vi "imp_test_v9_1.vi"() -> ()   [LabVIEW 2014]
uses:
  <vilib>/LabVIEW Targets/FPGA/cRIO/shared/nicrio_ModuleControls/nicrio_cRIO-9237_DataRatesRing.ctl
  <vilib>/LabVIEW Targets/FPGA/cRIO/shared/nicrio_ModuleControls/nicrio_cRIO-9237_ExcitationVoltageRing.ctl
  <vilib>/rvi/FXPMathLib/FxpSinAndCos/subVIs/nifxpmath_SinAndCos_SimConfig.ctl
  <vilib>/rvi/Emulation/niFpgaGetClockAttributes.vi
  <vilib>/rvi/Emulation/niFpgaSctlEmulationGetInTimedLoop.vi
  <vilib>/rvi/Emulation/niFpgaEmulationReportErrorSimple.vi
  <vilib>/rvi/Emulation/niFpgaProcessEmulError.vi
  <vilib>/rvi/interface/RandomDataEmulation/nirviRandomDataMultiElementFPGAFIFO.vi
  <instcachedir>/0/nirviRandomDataMultiElementFPGAFIFO_AD0CFC12EF974623A9C2E4184BC062B2.lvgen/nirviRandomDataMultiElementFPGAFIFO_AD0CFC12EF974623A9C2E4184BC062B2_025.vi
  <vilib>/rvi/interface/RandomDataEmulation/niFpgaRandomDataHandleErrors.vi
  <vilib>/rvi/Emulation/niFpgaCriticalErrorInLSC.vi
  <vilib>/rvi/FXPMathLib/FxpSinAndCos/simVIs/DllFxpSinAndCosTemp_sub.vi
  <vilib>/rvi/eio/common/nirviEmuTemplateMethod_errors.vi
  <vilib>/rvi/eio/common/nirviEmuTemplatePropertySet_errors.vi
  <vilib>/rvi/DataTransferAndStorage/Container/XNode/niFpgaContainer.xnode
  <vilib>/rvi/interface/RandomDataEmulation/nirviRandomDataFpgaMultiElementTemplate.vi
  <vilib>/rvi/FXPMathLib/FxpMul/XNode/nifxpmath_Multiplier.xnode
  <vilib>/rvi/FXPMathLib/FxpSinAndCos/XNode/nifxpmath_SinAndCos.xnode
  <vilib>/eio/EIONode/EIONode.xnode
  <vilib>/rvi/Analysis/measure/butterworth/XNode/niFpgaButterworthFilter.xnode
  <vilib>/rvi/FXPMathLib/FxpSub/XNode/nifxpmath_Sub.xnode
  <vilib>/rvi/FXPMathLib/FxpAdd/XNode/nifxpmath_Add.xnode
  <vilib>/eio/EIOPropertyNode/EIOPropertyNode.xnode
  <vilib>/rvi/eio/common/nirviEmuTemplatePropertyGet_errors.vi
  <vilib>/rvi/eio/common/nirviEmuTemplatePropertyGet_noerrors.vi
  <vilib>/rvi/eio/common/nirviEmuTemplatePropertySet_noerrors.vi
  <vilib>/rvi/FXPMathLib/sim/FxpSim.dll
panel:
  in  "Set 6":bool
  in  "Set 5":bool
  in  "Set 4":bool
  in  "Set 3":bool
  in  "Set 2":bool
  in  "Set 1":bool
  out "Dy1_d (T)":fxp<+/-,56,14>
  out "omega_y1 (T)":fxp<+/-,36,13>
  out "Dp1_d (T)":fxp<+/-,36,13>
  out "omega_p1 (T)":fxp<+/-,36,13>
  out "Dy2_d (T)":fxp<+/-,36,13>
  out "Dp2_d (T)":fxp<+/-,36,13>
  out "omega_y2 (T)":fxp<+/-,36,13>
  out "omega_p2 (T)":fxp<+/-,36,13>
  out "mt_omega_y2":u32
  out "mt_omega_p2":u32
  out "rad_y2":fxp<+/-,33,20>
  out "D_y2":fxp<+/-,32,7>
  out "rad_y1":fxp<+/-,33,20>
  out "D_y1":fxp<+/-,32,7>
  out "Encoder Position_y1":i32
  out "Encoder Position_y2":i32
  out "Encoder Position_p2":i32
  out "D_p2":fxp<+/-,32,7>
  out "rad_p2":fxp<+/-,33,20>
  out "D_p1":fxp<+/-,32,7>
  out "rad_p1":fxp<+/-,33,20>
  out "Encoder Position_p1":i32
  in  "Mag. factor_y":fxp<+/-,20,3>
  in  "Mag. encoder_y":bool
  out "omega_y (rad/s)":fxp<+/-,36,13>
  out "Dy_d (mm/s)":fxp<+/-,36,13>
  in  "Vy. Est.":i16(ring) items=["T", "Mavg"]
  out "omega_y (Mavg)":fxp<+/-,36,14>
  out "Dy_d (Mavg)":fxp<+/-,36,14>
  in  "Dy_d_M_avg_Tc (uSec)":i32
  out "Dp_d (Mavg)":fxp<+/-,36,14>
  out "omega_p (Mavg)":fxp<+/-,36,14>
  in  "Dp_d_M_avg_Tc (uSec)":i32
  out "Dp_d (T)":fxp<+/-,36,13>
  out "omega_p (T)":fxp<+/-,36,13>
  in  "Vp. Est.":i16(ring) items=["T", "Mavg"]
  in  "Mag. factor_p":fxp<+/-,20,3>
  in  "Mag. encoder_p":bool
  in  "Belt_out_p":fxp<+/-,7,7>
  in  "Belt_in_p":fxp<+/-,6,6>
  in  "Belt_out_y":fxp<+/-,7,7>
  in  "Belt_in_y":fxp<+/-,6,6>
  out "Fp_dc":fxp<+/-,32,10>
  out "Fy_dc":fxp<+/-,32,10>
  in  "Zero_y":bool
  in  "Zero_p":bool
  in  "mt0_omega_p":u32
  in  "Encoder reset":bool
  out "fpt_d":fxp<+/-,36,18>
  out "Dp_error_dd":fxp<+/-,36,16>
  out "Dp_error_d":fxp<+/-,33,8>
  in  "Dp_dd coeff.":i32[](array[numeric])=[946630756, 63555534]
  out "Dp_dd":fxp<+/-,36,25>
  out "dFp_PID":fxp<+/-,36,18>
  in  "dFp_PID coeff.":i32[](array[numeric])=[946630756, 63555534]
  out "fpt_i":fxp<+/-,34,18>
  in  "Bv_p":fxp<+/-,22,8>
  in  "Kv_p":fxp<+/-,22,8>
  out "Dp_error":fxp<+/-,22,7>
  out "Dpr_sin":fxp<+/-,22,7>
  in  "Sin offset_p":fxp<+/-,22,7>
  in  "Sin magnitude_p":fxp<+/-,21,6>
  out "Dpr_sin_dd":fxp<+/-,35,20>
  out "Dpr_sin_d":fxp<+/-,33,15>
  out "Sin omega_p":fxp<+/-,34,9>
  in  "Sin wave freq._p (Hz)":fxp<+/-,32,6>
  in  "Dpr_step":fxp<+/-,22,7>
  out "Dpr_for":fxp<+/-,22,7>
  in  "Command_p":i16(ring) items=["Step", "Sine"]
  in  "Ki_p":fxp<+/-,36,9>
  out "Fp_PID":fxp<+/-,36,16>
  in  "fp_tolorance":fxp<+,22,6>
  out "fp_tilde":fxp<+/-,33,10>
  in  "Kd_p":fxp<+/-,36,9>
  in  "Kp_p":fxp<+/-,36,9>
  out "Fr_p":fxp<+/-,32,10>
  in  "S/F coeff_p":fxp<+/-,25,-10>
  in  "S/F coeff_y":fxp<+/-,25,-10>
  out "va_p":fxp<+/-,36,7>
  out "vb_p":fxp<+/-,37,8>
  out "vq_p_F":fxp<+/-,20,5> format="%.57g"
  out "vd_p_F":fxp<+/-,20,5>
  in  "dFp_add":bool
  in  "Stop motor_p":bool
  out "Force_p":fxp<+/-,32,10>
  in  "Strain selection_p":i16(ring) items=["Raw", "Avg.8", "Avg.8 w. filter"]
  out "Strain_p (Avg8 w. f)":fxp<+/-,36,8>
  in  "Strain_p Avg.8 coeff.":i32[](array[numeric])=[946630756, 63555534]
  out "Strain_p (Avg8)":fxp<+/-,36,4>
  out "Raw Strain_p":fxp<+/-,36,4>
  out "Mod6/AI3":fxp<+/-,36,4>
  in  "Strain gage reset_p":bool
  out "Dp_d (mm/s)":fxp<+/-,36,13>
  out "omega_p (rad/s)":fxp<+/-,36,13>
  out "mt_omega_p1":u32
  out "rad_p(NrTheta)":fxp<+/-,33,20>
  out "D_p(mm)":fxp<+/-,32,7>
  out "Encoder Position_p":i32
  in  "Encoder reset_p":bool
  out "Strain_y (Avg8 w. f)":fxp<+/-,36,8>
  in  "Strain_y Avg8 coeff.":i32[](array[numeric])=[-898916953, 1957103773, 3888751]
  out "Dyr_for":fxp<+/-,22,7>
  in  "Command_y":i16(ring) items=["Step", "Sine"]
  out "Strain_y (Avg8)":fxp<+/-,36,4>
  in  "Strain selection_y":i16(ring) items=["Raw", "Avg.8", "Avg.8 w. filter"]
  out "vb_y":fxp<+/-,38,8>
  out "va_y":fxp<+/-,38,8>
  out "fyt_d":fxp<+/-,36,18>
  out "Fr_y":fxp<+/-,32,10>
  in  "Bv_y":fxp<+/-,22,8>
  out "Dy_error_dd":fxp<+/-,36,16>
  out "Dy_error_d":fxp<+/-,33,8>
  in  "Kv_y":fxp<+/-,22,8>
  out "Dy_error":fxp<+/-,22,7>
  out "Dyr_sin_dd":fxp<+/-,35,20>
  out "Dyr_sin_d":fxp<+/-,33,15>
  out "Sin omega_y":fxp<+/-,34,9>
  out "Dyr_sin":fxp<+/-,22,7>
  in  "Sin offset_y":fxp<+/-,22,7>
  in  "Sin magnitude_y":fxp<+/-,21,6>
  out "Time now(s)":fxp<+,52,14>
  in  "Sin wave freq._y (Hz)":fxp<+/-,32,6>
  in  "Dyr_step":fxp<+/-,22,7>
  in  "Drive mode":i16(ring) items=["Backward", "Forward"]
  out "Dy_dd":fxp<+/-,36,25>
  in  "Dy_dd coeff.":i32[](array[numeric])=[946630756, 63555534]
  out "dFy_PID":fxp<+/-,36,18>
  in  "dFy_PID coeff.":i32[](array[numeric])=[946630756, 63555534]
  out "fyt_i":fxp<+/-,36,16>
  out "Fy_PID":fxp<+/-,36,16>
  in  "fy_tolorance":fxp<+,22,6>
  in  "Ki_y":fxp<+/-,36,9>
  in  "Kd_y":fxp<+/-,36,9>
  out "fy_tilde":fxp<+/-,32,10>
  in  "Kp_y":fxp<+/-,36,9>
  out "vq_y_F":fxp<+/-,20,5> format="%.57g"
  out "vd_y_F":fxp<+/-,20,5>
  in  "dFy_add":bool
  in  "Stop motor_y":bool
  out "Dy_d (T)":fxp<+/-,36,13>
  out "omega_y (T)":fxp<+/-,36,13>
  in  "mt0_omega_y":u32
  out "mt_omega_y1":u32
  out "rad_y(NrTheta)":fxp<+/-,33,20>
  out "D_y(mm)":fxp<+/-,32,7>
  out "Encoder Position_y":i32
  in  "Encoder reset_y":bool
  in  "Ini coe.":bool
  out "Loop rate (kHz)":fxp<+/-,36,7>
  out "Force_y":fxp<+/-,32,10>
  out "Raw Strain_y":fxp<+/-,36,4>
  in  "Strain gage reset_y":bool
  in  "Stop (Strain)":bool
  out "Mod6/AI2":fxp<+/-,36,4>
  in  "Excitation Voltage":T1 items=["2.5 Volts", "3.3 Volts", "5.0 Volts", "10.0 Volts", "External Excitation"]
  in  "Data Rate":T2=1 items=["50.000 kS/s (NI 9237)"=1, "25.000 kS/s (NI 9237)"=2, "16.667 kS/s (NI 9237)"=3, "12.500 kS/s (NI 9237)"=4, "10.000 kS/s (NI 9237)"=5, "8.333 kS/s (NI 9237)"=6, "7.143 kS/s (NI 9237)"=7, "6.250 kS/s (NI 9237)"=8, "5.556 kS/s (NI 9237)"=9, "5.000 kS/s (NI 9237)"=10, "4.545 kS/s (NI 9237)"=11, "4.167 kS/s (NI 9237)"=12, "3.846 kS/s (NI 9237)"=13, "3.571 kS/s (NI 9237)"=14, "3.333 kS/s (NI 9237)"=15, "3.125 kS/s (NI 9237)"=16, "2.941 kS/s (NI 9237)"=17, "2.778 kS/s (NI 9237)"=18, "2.632 kS/s (NI 9237)"=19, "2.500 kS/s (NI 9237)"=20, "2.381 kS/s (NI 9237)"=21, "2.273 kS/s (NI 9237)"=22, "2.174 kS/s (NI 9237)"=23, "2.083 kS/s (NI 9237)"=24, "2.000 kS/s (NI 9237)"=25, "1.923 kS/s (NI 9237)"=26, "1.852 kS/s (NI 9237)"=27, "1.786 kS/s (NI 9237)"=28, "1.724 kS/s (NI 9237)"=29, "1.667 kS/s (NI 9237)"=30, "1.613 kS/s (NI 9237)"=31]
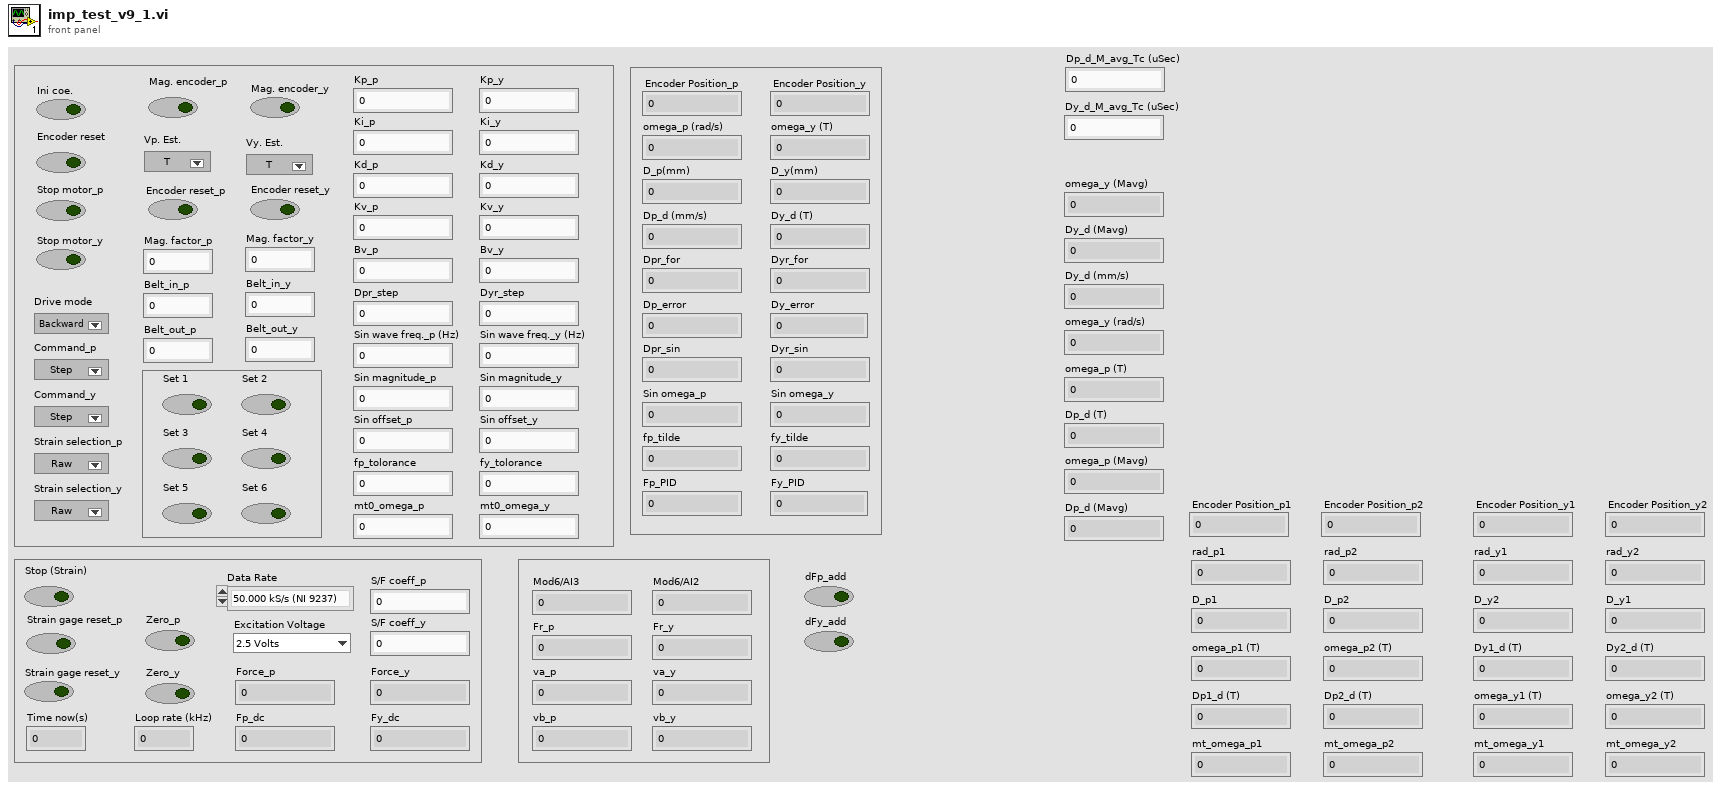
[diagram p1: front panel]
types:
  T1 = typedef "nicrio_cRIO-9237_ExcitationVoltageRing.ctl" = u8
  T2 = typedef "nicrio_cRIO-9237_DataRatesRing.ctl" = u8
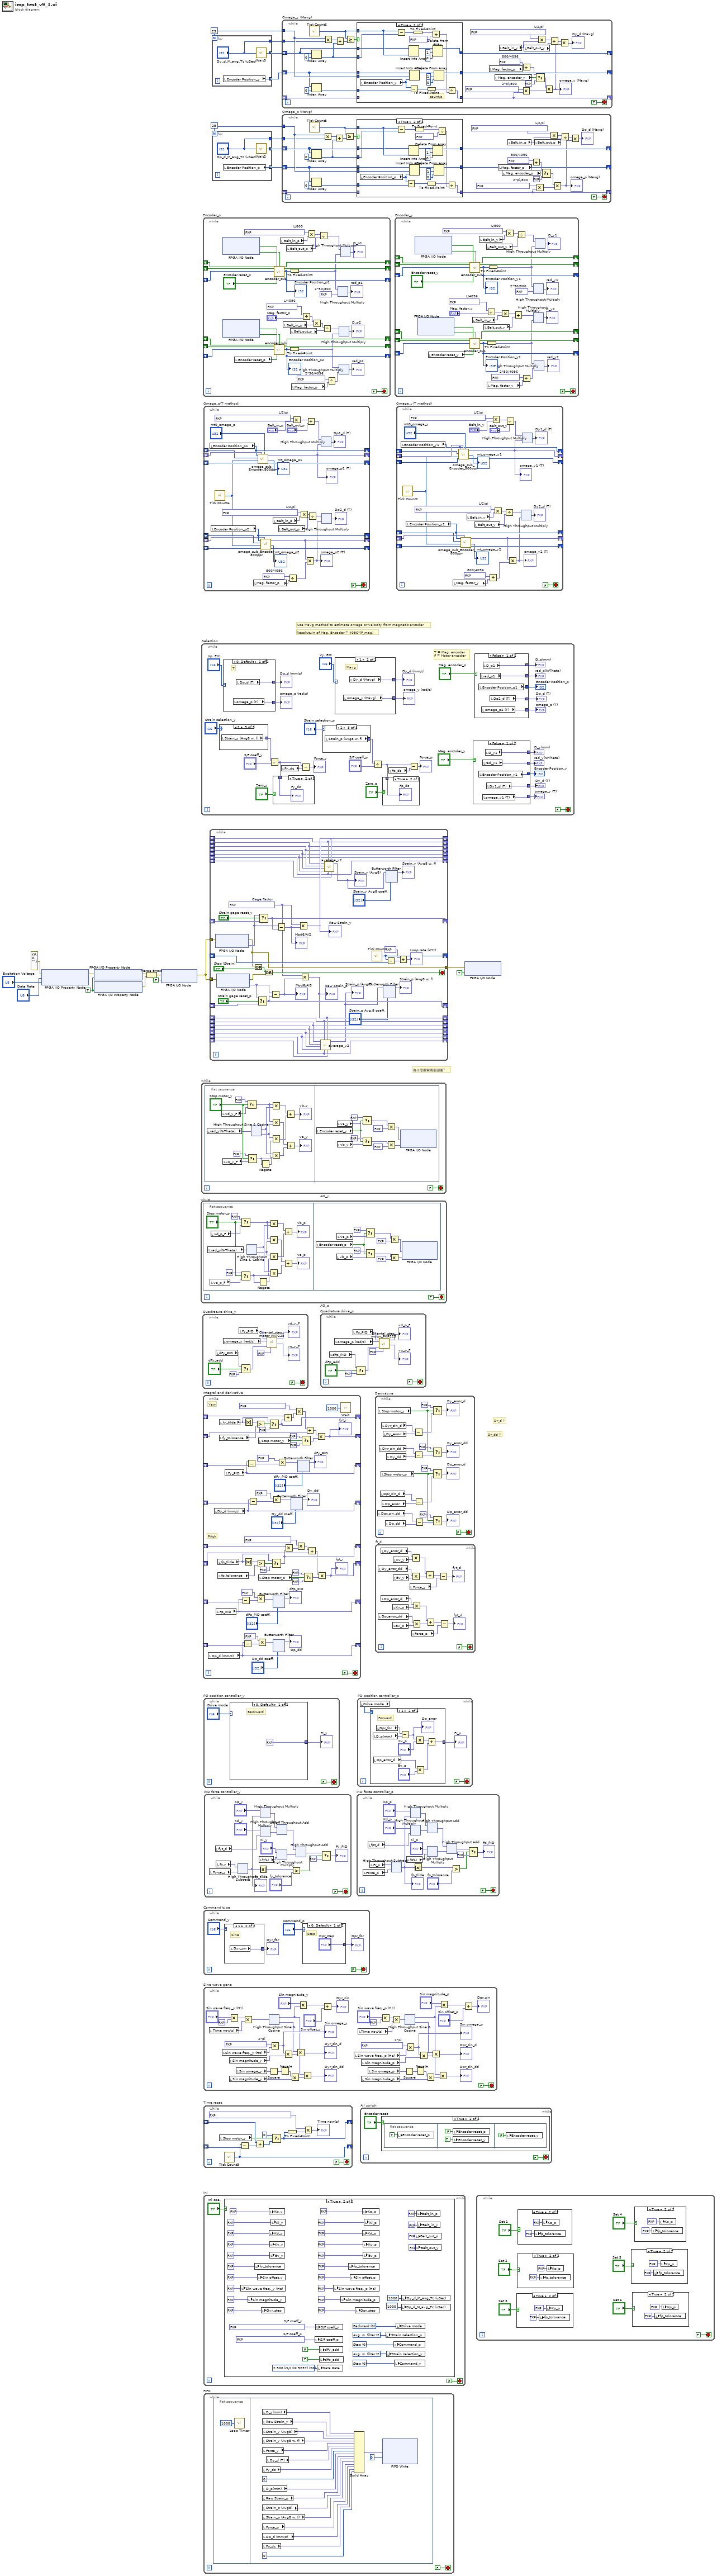
[diagram p0: block diagram]
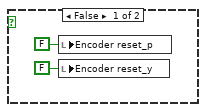
[diagram p10: hidden frame]
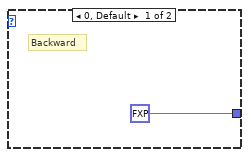
[diagram p11: hidden frame]
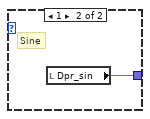
[diagram p12: hidden frame]
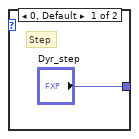
[diagram p13: hidden frame]
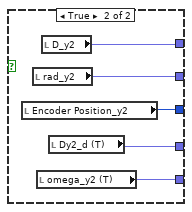
[diagram p14: hidden frame]
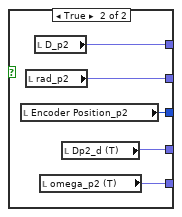
[diagram p15: hidden frame]
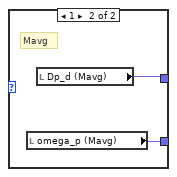
[diagram p16: hidden frame]
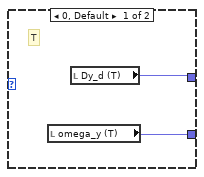
[diagram p17: hidden frame]
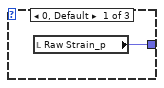
[diagram p20: hidden frame]
diagram:
  w5 = 25
  w8 = 25
  w13 = TRUE ("Half-Bridge Enable")
  # "Resolutuin of Mag. Encoder = 4096*(F_mag)"
  # "use Mavg method to estimate omega or velocity from magnetic encoder"
  # "為什麼要寫兩個迴圈?"
  # "Dr_dd ?"
  # "Dr_d ?"
  n1 = xnode "FPGA I/O Property Node"("error in"=errorcluster {"status"=FALSE, "code"=0, "source"=""}, "Data Rate"="Data Rate", "Excitation Voltage"="Excitation Voltage") -> ("error out"=w18:errorcluster)  [unwired: 1 in, 1 out]
  n2 = xnode "FPGA I/O Property Node"("error in"=w18, "Half-Bridge Enable"=w13) -> ("error out"=w11:errorcluster)  [unwired: 1 in, 1 out]
  n3 = xnode "FPGA I/O Property Node"("Half-Bridge Enable"=w13) -> ("error out"=w10:errorcluster)  [unwired: 2 in, 1 out]
  n4 = Merge Errors(w11, w10) -> (w12:errorcluster)
  n5 = xnode "FPGA I/O Node"("error in"=w12, "Mod6/Start"=TRUE) -> ("error out"=w16:errorcluster)  [unwired: 1 in, 1 out]
  n6 = while "AO_p" {
    stop <- FALSE stop-if-true
    n7 = flat-sequence {
      frame #0 {
        n8 = local read "rad_p(NrTheta)"() -> (w33:fxp<+/-,33,20>)
        n9 = local read "vq_p_F"() -> (w34:fxp<+/-,20,5>)
        n10 = local read "vd_p_F"() -> (w36:fxp<+/-,20,5>)
        n11 = Select(t=fxp<+/-,20,5> 0.0, s="Stop motor_p", f=w36) -> (s? t:f=w25:fxp<+/-,20,5>)
        n12 = Select(t=fxp<+,1,1> 0.0, s="Stop motor_p", f=w34) -> (s? t:f=w24:fxp<+/-,20,5>)
        n13 = xnode "High Throughput Sine & Cosine"("x (pi)"=w33) -> ("sin(x)"=w27:fxp<+/-,16,2>, "cos(x)"=w26:fxp<+/-,16,2>)
        n14 = Negate(x=w24) -> (-x=w32:fxp<+/-,21,6>)
        n15 = Multiply(x=w25, y=w27) -> (x*y=w31:fxp<+/-,36,7>)
        n16 = Multiply(x=w25, y=w26) -> (x*y=w29:fxp<+/-,36,7>)
        n17 = Multiply(x=w26, y=w24) -> (x*y=w30:fxp<+/-,36,7>)
        n18 = Multiply(x=w27, y=w32) -> (x*y=w28:fxp<+/-,35,6>)
        n19 = Add(x=w31, y=w30) -> (x+y=→"vb_p":fxp<+/-,37,8>)
        n20 = Add(x=w29, y=w28) -> (x+y=→"va_p":fxp<+/-,36,7>)
      }
      frame #1 {
        n21 = local read "Encoder reset_p"() -> (w69:bool)
        n22 = local read "vb_p"() -> (w70:fxp<+/-,37,8>)
        n23 = local read "va_p"() -> (w71:fxp<+/-,36,7>)
        n24 = Select(t=fxp<+,2,2> 3.0, s=w69, f=w71) -> (s? t:f=w77:fxp<+/-,36,7>)
        n25 = Select(t=fxp<+,1,1> 0.0, s=w69, f=w70) -> (s? t:f=w76:fxp<+/-,37,8>)
        n26 = Multiply(x=w77, y=fxp<+/-,1,0> -0.5) -> (x*y=w72:fxp<+/-,36,6>)
        n27 = Multiply(x=w76, y=fxp<+/-,1,0> -0.5) -> (x*y=w73:fxp<+/-,36,6>)
        n28 = xnode "FPGA I/O Node"("Mod8/AO0"=w72, "Mod8/AO1"=w73) -> ()  [unwired: 2 in, 2 out]
      }
    }
  }
  n29 = while "AO_y" {
    stop <- FALSE stop-if-true
    n30 = flat-sequence {
      frame #0 {
        n31 = local read "rad_y(NrTheta)"() -> (w97:fxp<+/-,33,20>)
        n32 = local read "vd_y_F"() -> (w95:fxp<+/-,20,5>)
        n33 = local read "vq_y_F"() -> (w94:fxp<+/-,20,5>)
        n34 = Select(t=fxp<+/-,20,5> 0.0, s="Stop motor_y", f=w95) -> (s? t:f=w89:fxp<+/-,20,5>)
        n35 = Select(t=fxp<+/-,20,5> 0.0, s="Stop motor_y", f=w94) -> (s? t:f=w88:fxp<+/-,20,5>)
        n36 = xnode "High Throughput Sine & Cosine"("x (pi)"=w97) -> ("sin(x)"=w91:fxp<+/-,17,2>, "cos(x)"=w90:fxp<+/-,17,2>)
        n37 = Negate(x=w88) -> (-x=w87:fxp<+/-,21,6>)
        n38 = Multiply(x=w89, y=w91) -> (x*y=w86:fxp<+/-,37,7>)
        n39 = Multiply(x=w89, y=w90) -> (x*y=w84:fxp<+/-,37,7>)
        n40 = Multiply(x=w90, y=w88) -> (x*y=w85:fxp<+/-,37,7>)
        n41 = Multiply(x=w91, y=w87) -> (x*y=w83:fxp<+/-,36,6>)
        n42 = Add(x=w86, y=w85) -> (x+y=→"vb_y":fxp<+/-,38,8>)
        n43 = Add(x=w84, y=w83) -> (x+y=→"va_y":fxp<+/-,37,7>)
      }
      frame #1 {
        n44 = local read "Encoder reset_y"() -> (w130:bool)
        n45 = local read "va_y"() -> (w129:fxp<+/-,38,8>)
        n46 = local read "vb_y"() -> (w128:fxp<+/-,38,8>)
        n47 = Select(t=fxp<+,2,2> 3.0, s=w130, f=w129) -> (s? t:f=w134:fxp<+/-,38,8>)
        n48 = Select(t=fxp<+,1,1> 0.0, s=w130, f=w128) -> (s? t:f=w133:fxp<+/-,38,8>)
        n49 = Multiply(x=w134, y=fxp<+/-,1,0> -0.5) -> (x*y=w137:fxp<+/-,39,8>)
        n50 = Multiply(x=w133, y=fxp<+/-,1,0> -0.5) -> (x*y=w138:fxp<+/-,37,6>)
        n51 = xnode "FPGA I/O Node"("Mod8/AO2"=w137, "Mod8/AO3"=w138) -> ()  [unwired: 2 in, 2 out]
      }
    }
  }
  n52 = while "Selection" {
    stop <- FALSE stop-if-true
    # "T = Mag. encoder\nF = Motor encoder"
    n53 = case shown="2" "Strain selection_y" {
      tunnel: [w205 w206 w207] -> w170
      frame 0, Default {
        n54 = local read "Raw Strain_y"() -> (w205:fxp<+/-,36,4>)
      }
      frame 1 {
        n55 = local read "Strain_y (Avg8)"() -> (w206:fxp<+/-,36,4>)
      }
      frame 2 {
        n56 = local read "Strain_y (Avg8 w. f)"() -> (w207:fxp<+/-,36,8>)
      }
    }
    n57 = case shown="0, Default" "Vp. Est." {
      tunnel: [w193 w194] -> w153
      tunnel: [w192 w195] -> w154
      frame 0, Default {
        # "T"
        n58 = local read "omega_p (T)"() -> (w193:fxp<+/-,36,13>)
        n59 = local read "Dp_d (T)"() -> (w192:fxp<+/-,36,13>)
      }
      frame 1 {
        # "Mavg"
        n60 = local read "omega_p (Mavg)"() -> (w194:fxp<+/-,36,14>)
        n61 = local read "Dp_d (Mavg)"() -> (w195:fxp<+/-,36,14>)
      }
    }
    "Dp_d (mm/s)" <- w154
    "omega_p (rad/s)" <- w153
    n62 = Divide(x=w170, y="S/F coeff_y") -> (x/y=w163:fxp<+/-,32,10>)
    n63 = case shown="True" "Zero_y" {
      tunnel: w163 -> [_ w201]
      frame False {
      }
      frame True {
        "Fy_dc" <- w201
      }
    }
    n64 = local read "Fy_dc"() -> (w164:fxp<+/-,32,10>)
    n65 = Subtract(x=w163, y=w164) -> (x-y=→"Force_y":fxp<+/-,33,11>)
    n66 = case shown="2" "Strain selection_p" {
      tunnel: [w202 w203 w204] -> w168
      frame 0, Default {
        n67 = local read "Raw Strain_p"() -> (w202:fxp<+/-,36,4>)
      }
      frame 1 {
        n68 = local read "Strain_p (Avg8)"() -> (w203:fxp<+/-,36,4>)
      }
      frame 2 {
        n69 = local read "Strain_p (Avg8 w. f)"() -> (w204:fxp<+/-,36,8>)
      }
    }
    n70 = case shown="1" "Vy. Est." {
      tunnel: [w197 w199] -> w156
      tunnel: [w196 w198] -> w157
      frame 0, Default {
        # "T"
        n71 = local read "omega_y (T)"() -> (w196:fxp<+/-,36,13>)
        n72 = local read "Dy_d (T)"() -> (w197:fxp<+/-,36,13>)
      }
      frame 1 {
        # "Mavg"
        n73 = local read "omega_y (Mavg)"() -> (w198:fxp<+/-,36,14>)
        n74 = local read "Dy_d (Mavg)"() -> (w199:fxp<+/-,36,14>)
      }
    }
    "Dy_d (mm/s)" <- w156
    "omega_y (rad/s)" <- w157
    n75 = Divide(x=w168, y="S/F coeff_p") -> (x/y=w160:fxp<+/-,32,10>)
    n76 = case shown="True" "Zero_p" {
      tunnel: w160 -> [_ w200]
      frame False {
      }
      frame True {
        "Fp_dc" <- w200
      }
    }
    n77 = local read "Fp_dc"() -> (w158:fxp<+/-,32,10>)
    n78 = Subtract(x=w160, y=w158) -> (x-y=→"Force_p":fxp<+/-,33,11>)
    n79 = case shown="False" "Mag. encoder_y" {
      tunnel: [w176 w180] -> w144
      tunnel: [w175 w181] -> w145
      tunnel: [w174 w179] -> w147
      tunnel: [w172 w178] -> w141
      tunnel: [w173 w177] -> w140
      frame False {
        n80 = local read "Encoder Position_y1"() -> (w174:i32)
        n81 = local read "rad_y1"() -> (w176:fxp<+/-,33,20>)
        n82 = local read "omega_y1 (T)"() -> (w172:fxp<+/-,36,13>)
        n83 = local read "D_y1"() -> (w175:fxp<+/-,32,7>)
        n84 = local read "Dy1_d (T)"() -> (w173:fxp<+/-,56,14>)
      }
      frame True {
        n85 = local read "Encoder Position_y2"() -> (w179:i32)
        n86 = local read "rad_y2"() -> (w180:fxp<+/-,33,20>)
        n87 = local read "omega_y2 (T)"() -> (w178:fxp<+/-,36,13>)
        n88 = local read "D_y2"() -> (w181:fxp<+/-,32,7>)
        n89 = local read "Dy2_d (T)"() -> (w177:fxp<+/-,36,13>)
      }
    }
    "D_y(mm)" <- w145
    "rad_y(NrTheta)" <- w144
    "Encoder Position_y" <- w147
    "Dy_d (T)" <- w140
    "omega_y (T)" <- w141
    n90 = case shown="False" "Mag. encoder_p" {
      tunnel: [w186 w191] -> w149
      tunnel: [w185 w190] -> w150
      tunnel: [w184 w189] -> w151
      tunnel: [w182 w188] -> w143
      tunnel: [w183 w187] -> w142
      frame False {
        n91 = local read "Encoder Position_p1"() -> (w184:i32)
        n92 = local read "rad_p1"() -> (w185:fxp<+/-,33,20>)
        n93 = local read "omega_p2 (T)"() -> (w182:fxp<+/-,36,13>)
        n94 = local read "D_p1"() -> (w186:fxp<+/-,32,7>)
        n95 = local read "Dp2_d (T)"() -> (w183:fxp<+/-,36,13>)
      }
      frame True {
        n96 = local read "Encoder Position_p2"() -> (w189:i32)
        n97 = local read "rad_p2"() -> (w190:fxp<+/-,33,20>)
        n98 = local read "D_p2"() -> (w191:fxp<+/-,32,7>)
        n99 = local read "omega_p2 (T)"() -> (w188:fxp<+/-,36,13>)
        n100 = local read "Dp2_d (T)"() -> (w187:fxp<+/-,36,13>)
      }
    }
    "D_p(mm)" <- w149
    "rad_p(NrTheta)" <- w150
    "Encoder Position_p" <- w151
    "Dp_d (T)" <- w142
    "omega_p (T)" <- w143
  }
  n101 = while "Quadrature drive_y" {
    stop <- FALSE stop-if-true
    n102 = local read "dFy_PID"() -> (w209:fxp<+/-,36,18>)
    n103 = local read "omega_y (rad/s)"() -> (w217:fxp<+/-,36,13>)
    n104 = local read "Fy_PID"() -> (w210:fxp<+/-,36,16>)
    n105 = Select(t=w209, s="dFy_add", f=fxp<+,1,1> 0.0) -> (s? t:f=w213:fxp<+/-,36,18>)
    n106 = call "Oriental_step_motor_PKP225.vi"("F_Threshold"=fxp<+,12,12> 10.0, "dFmr"=w213, "omega"=w217, "Fmr"=w210) -> ("vq_F"=→"vq_y_F":fxp<+/-,20,5>, "vd_F"=→"vd_y_F":fxp<+/-,20,5>)  [unwired: 6 in]
  }
  n107 = while "Encoder_p" {
    shift-right: [w255] -> _
    shift-left: _ -> [w254]
    shift-right: [w256] -> _
    shift-left: _ -> [w253]
    shift-right: [w250] -> _
    shift-left: _ -> [w252]
    shift-right: [w236] -> _
    shift-left: _ -> [w235]
    shift-right: [w237] -> _
    shift-left: _ -> [w238]
    shift-right: [w232] -> _
    shift-left: _ -> [w233]
    stop <- FALSE stop-if-true
    w225 = fxp<+/-,20,-5> 0.00048828125  # L/4096
    w221 = fxp<+/-,16,1> 0.0244140625  # 2*50/4096
    w245 = fxp<+/-,20,-5> 0.002499997615814209  # L/800
    w249 = fxp<+/-,16,1> 0.125  # 2*50/800
    n108 = xnode "FPGA I/O Node"() -> ("Mod7/DIO0"=w258:bool, "Mod7/DIO1"=w257:bool)  [unwired: 2 in, 2 out]
    n109 = xnode "FPGA I/O Node"() -> ("Mod7/DIO4"=w240:bool, "Mod7/DIO5"=w239:bool)  [unwired: 2 in, 2 out]
    n110 = local read "Encoder reset_p"() -> (w234:bool)
    n111 = call "encoder_sub.vi"("A_pre"=w254, "B_pre"=w253, "Encoder Position_pre"=w252, "A input"=w258, "Encoder Position Reset"="Encoder reset_p", "B input"=w257) -> ("A"=w255:bool, "B"=w256:bool, "Encoder Position (Counts)"=w250:i32)  [unwired: 19 in]
    "Encoder Position_p1" <- w250
    n112 = call "encoder_sub.vi"("A_pre"=w235, "B_pre"=w238, "Encoder Position_pre"=w233, "A input"=w240, "Encoder Position Reset"=w234, "B input"=w239) -> ("A"=w236:bool, "B"=w237:bool, "Encoder Position (Counts)"=w232:i32)  [unwired: 19 in]
    "Encoder Position_p2" <- w232
    n113 = local read "Belt_in_p"() -> (w244:fxp<+/-,6,6>)
    n114 = local read "Belt_in_p"() -> (w226:fxp<+/-,6,6>)
    n115 = local read "Belt_out_p"() -> (w242:fxp<+/-,7,7>)
    n116 = To Fixed-Point(number=w232) -> (fixed-point=w229:fxp<+/-,21,21>)  [unwired: 1 in]
    n117 = To Fixed-Point(number=w250) -> (fixed-point=w247:fxp<+/-,16,16>)  [unwired: 1 in]
    n118 = local read "Belt_out_p"() -> (w228:fxp<+/-,7,7>)
    n119 = local read "Mag. factor_p"() -> (w220:fxp<+/-,20,3>)
    n120 = Divide(x=w225, y="Mag. factor_p") -> (x/y=w224:fxp<+/-,32,0>)
    n121 = Multiply(x=w245, y=w244) -> (x*y=w243:fxp<+/-,26,1>)
    n122 = Multiply(x=w224, y=w226) -> (x*y=w227:fxp<+/-,32,6>)
    n123 = Divide(x=w243, y=w242) -> (x/y=w241:fxp<+/-,27,2>)
    n124 = Divide(x=w227, y=w228) -> (x/y=w223:fxp<+/-,36,6>)
    n125 = Divide(x=w221, y=w220) -> (x/y=w222:fxp<+/-,20,0>)
    n126 = xnode "High Throughput Multiply"("x"=w247, "y"=w249) -> ("x*y"=→"rad_p1":fxp<+/-,32,17>)
    n127 = xnode "High Throughput Multiply"("x"=w223, "y"=w229) -> ("x*y"=→"D_p2":fxp<+/-,57,27>)
    n128 = xnode "High Throughput Multiply"("x"=w229, "y"=w222) -> ("x*y"=→"rad_p2":fxp<+/-,41,21>)
    n129 = xnode "High Throughput Multiply"("x"=w241, "y"=w247) -> ("x*y"=→"D_p1":fxp<+/-,43,18>)
  }
  n130 = while "Integral and derivative" {
    shift-right: [w314] -> _
    shift-left: _ -> [w313]
    shift-right: [w306] -> _
    shift-left: _ -> [w305]
    shift-right: [w316] -> _
    shift-left: _ -> [w317]
    shift-right: [w296] -> _
    shift-left: _ -> [w295]
    shift-right: [w282] -> _
    shift-left: _ -> [w285]
    shift-right: [w275] -> _
    shift-left: _ -> [w274]
    shift-right: [w269] -> _
    shift-left: _ -> [w268]
    shift-right: [w264] -> _
    shift-left: _ -> [w265]
    stop <- FALSE stop-if-true
    # "Pitch"
    # "Yaw"
    n131 = local read "Dp_d (mm/s)"() -> (w264:fxp<+/-,36,13>)
    n132 = local read "Dy_d (mm/s)"() -> (w296:fxp<+/-,36,13>)
    n133 = local read "Fp_PID"() -> (w269:fxp<+/-,36,16>)
    n134 = local read "fp_tilde"() -> (w286:fxp<+/-,33,10>)
    n135 = local read "fp_tolorance"() -> (w289:fxp<+,22,6>)
    n136 = local read "fy_tolorance"() -> (w292:fxp<+,22,6>)
    n137 = local read "fy_tilde"() -> (w318:fxp<+/-,32,10>)
    n138 = local read "Fy_PID"() -> (w316:fxp<+/-,36,16>)
    n139 = Subtract(x=w269, y=w268) -> (x-y=w273:fxp<+/-,37,17>)
    n140 = Subtract(x=w264, y=w265) -> (x-y=w266:fxp<+/-,37,14>)
    n141 = Absolute Value(x=w286) -> (abs(x)=w290:fxp<+,33,10>)
    n142 = Absolute Value(x=w318) -> (abs(x)=w320:fxp<+,32,10>)
    n143 = Subtract(x=w316, y=w317) -> (x-y=w304:fxp<+/-,37,17>)
    n144 = Subtract(x=w296, y=w295) -> (x-y=w298:fxp<+/-,36,11>)
    n145 = Greater?(x=w320, y=w292) -> (0:w321:bool)
    n146 = Greater?(x=w290, y=w289) -> (0:w288:bool)
    n147 = Multiply(x=fxp<+,7,10> 1000.0, y=w273) -> (x*y=w271:fxp<+/-,32,18>)
    n148 = Multiply(x=fxp<+,7,10> 1000.0, y=w266) -> (x*y=w262:fxp<+/-,36,21>)
    n149 = local read "Stop motor_y"() -> (w307:bool)
    n150 = local read "Stop motor_p"() -> (w277:bool)
    n151 = Select(t=w318, s=w321, f=fxp<+/-,33,11> 0.0) -> (s? t:f=w314:fxp<+/-,33,11>)
    n152 = Select(t=w286, s=w288, f=fxp<+,1,1> 0.0) -> (s? t:f=w282:fxp<+/-,33,10>)
    n153 = Multiply(x=fxp<+,7,10> 1000.0, y=w298) -> (x*y=w297:fxp<+/-,36,21>)
    n154 = xnode "Butterworth Filter"("input data"=w271, "scaled coefficients"="dFp_PID coeff.") -> ("output data"=→"dFp_PID":fxp<+/-,36,22>)  [unwired: 1 in]
    n155 = xnode "Butterworth Filter"("input data"=w262, "scaled coefficients"="Dp_dd coeff.") -> ("output data"=→"Dp_dd":fxp<+/-,36,25>)  [unwired: 1 in]
    n156 = Multiply(x=fxp<+,7,10> 1000.0, y=w304) -> (x*y=w301:fxp<+/-,32,18>)
    n157 = Add(x=w313, y=w314) -> (x+y=w319:fxp<+/-,34,12>)
    n158 = Multiply(x=w285, y=w282) -> (x*y=w284:fxp<+/-,34,12>)
    n159 = xnode "Butterworth Filter"("input data"=w297, "scaled coefficients"="Dy_dd coeff.") -> ("output data"=→"Dy_dd":fxp<+/-,36,25>)  [unwired: 1 in]
    n160 = Multiply(x=fxp<+/-,30,12> 0.000499725341796875, y=w319) -> (x*y=w312:fxp<+/-,34,10>)
    n161 = Multiply(x=fxp<+/-,30,12> 0.000499725341796875, y=w284) -> (x*y=w281:fxp<+/-,34,10>)
    n162 = xnode "Butterworth Filter"("input data"=w301, "scaled coefficients"="dFy_PID coeff.") -> ("output data"=→"dFy_PID":fxp<+/-,36,22>)  [unwired: 1 in]
    n163 = Select(t=fxp<+,1,1> 0.0, s=w307, f=fxp<+,1,1> 1.0) -> (s? t:f=w310:fxp<+,1,1>)
    n164 = Select(t=fxp<+,1,1> 0.0, s=w277, f=fxp<+,1,1> 1.0) -> (s? t:f=w279:fxp<+,1,1>)
    n165 = Add(x=w312, y=w305) -> (x+y=w311:fxp<+/-,36,16>)
    n166 = Add(x=w281, y=w274) -> (x+y=w280:fxp<+/-,36,16>)
    n167 = Multiply(x=w311, y=w310) -> (x*y=w306:fxp<+/-,34,18>)
    "fyt_i" <- w306
    n168 = Multiply(x=w280, y=w279) -> (x*y=w275:fxp<+/-,34,18>)
    "fpt_i" <- w275
    n169 = call "Wait"("Count(uSec)"=u32 1000) -> ()  [unwired: 1 out]
  }
  n170 = while "Omega_p(T method)" {
    shift-right: [w387] -> _
    shift-left: _ -> [w385]
    shift-right: [w366] -> _
    shift-left: _ -> [w386]
    shift-right: [w383] -> _
    shift-left: _ -> [w384]
    shift-right: [w373] -> _
    shift-left: _ -> [w372]
    shift-right: [w365] -> _
    shift-left: _ -> [w371]
    shift-right: [w370] -> _
    shift-left: _ -> [w369]
    stop <- FALSE stop-if-true
    w362 = fxp<+/-,32,0> 0.3183098859153688  # L/2/pi
    w375 = fxp<+,32,0> 0.1953125  # 800/4096
    w380 = fxp<+/-,32,0> 0.3183098859153688  # L/2/pi
    n171 = local read "Encoder Position_p1"() -> (w387:i32)
    n172 = local read "Encoder Position_p2"() -> (w373:i32)
    n173 = call "Tick Count4"() -> ("Tick Count(Ticks)"=w368:u32)
    n174 = local read "Mag. factor_p"() -> (w374:fxp<+/-,20,3>)
    n175 = call "omega_sub_Encoder_800ppr.vi"("mt0"="mt0_omega_p", "omega_pre"=w386, "ticks_m_pre"=w384, "ticks"=w368, "count_pre"=w385, "count"=w387) -> ("ticks_m"=w383:u32, "mt"=→"mt_omega_p1":u32, "omega"=w366:fxp<+/-,36,13>)  [unwired: 3 in]
    "omega_p1 (T)" <- w366
    n176 = call "omega_sub_Encoder_800ppr.vi"("omega_pre"=w371, "ticks_m_pre"=w369, "ticks"=w368, "count_pre"=w372, "count"=w373) -> ("ticks_m"=w370:u32, "mt"=→"mt_omega_p2":u32, "omega"=w365:fxp<+/-,36,13>)  [unwired: 4 in]
    n177 = local read "Belt_in_p"() -> (w359:fxp<+/-,6,6>)
    n178 = local read "Belt_out_p"() -> (w358:fxp<+/-,7,7>)
    n179 = Divide(x=w375, y=w374) -> (x/y=w364:fxp<+/-,53,18>)
    n180 = Multiply(x=w380, y="Belt_in_p") -> (x*y=w378:fxp<+/-,38,6>)
    n181 = Multiply(x=w362, y=w359) -> (x*y=w361:fxp<+/-,38,6>)
    n182 = Multiply(x=w365, y=w364) -> (x*y=w363:fxp<+/-,64,30>)
    "omega_p2 (T)" <- w363
    n183 = Divide(x=w378, y="Belt_out_p") -> (x/y=w376:fxp<+/-,20,1>)
    n184 = Divide(x=w361, y=w358) -> (x/y=w360:fxp<+/-,45,6>)
    n185 = xnode ("High Throughput Multiply")("x"=w376, "y"=w366) -> ("x*y"=→"Dp1_d (T)":fxp<+/-,56,14>)
    n186 = xnode ("High Throughput Multiply")("x"=w360, "y"=w363) -> ("x*y"=→"Dp2_d (T)":fxp<+/-,64,36>)
  }
  n187 = while "PD position controller_y" {
    stop <- FALSE stop-if-true
    n188 = case shown="0, Default" "Drive mode" {
      tunnel: [fxp<+/-,62,19> 0.0 w393] -> w389
      frame 0, Default {
        # "Backward"
      }
      frame 1 {
        # "Forward"
        n189 = local read "Dy_error_d"() -> (w395:fxp<+/-,33,8>)
        n190 = local read "D_y(mm)"() -> (w400:fxp<+/-,32,7>)
        n191 = local read "Dyr_for"() -> (w392:fxp<+/-,22,7>)
        n192 = Subtract(x=w392, y=w400) -> (x-y=w399:fxp<+/-,33,8>)
        "Dy_error" <- w399
        n193 = Multiply(x=w399, y="Kv_y") -> (x*y=w397:fxp<+/-,54,15>)
        n194 = Multiply(x=w395, y="Bv_y") -> (x*y=w394:fxp<+/-,55,16>)
        n195 = Add(x=w397, y=w394) -> (x+y=w393:fxp<+/-,55,16>)
      }
    }
    "Fr_y" <- w389
  }
  n196 = while "Command type" {
    stop <- FALSE stop-if-true
    n197 = case shown="1" "Command_y" {
      tunnel: ["Dyr_step" w409] -> w404
      frame 0, Default {
        # "Step"
      }
      frame 1 {
        # "Sine"
        n198 = local read "Dyr_sin"() -> (w409:fxp<+/-,22,7>)
      }
    }
    "Dyr_for" <- w404
    n199 = case shown="0, Default" "Command_p" {
      tunnel: ["Dpr_step" w407] -> w402
      frame 0, Default {
        # "Step"
      }
      frame 1 {
        # "Sine"
        n200 = local read "Dpr_sin"() -> (w407:fxp<+/-,22,7>)
      }
    }
    "Dpr_for" <- w402
  }
  n201 = while "Sine wave gene" {
    stop <- FALSE stop-if-true
    w415 = fxp<+,20,3> 6.2831878662109375  # 2*pi
    w447 = fxp<+,20,3> 6.2831878662109375  # 2*pi
    n202 = local read "Time now(s)"() -> (w453:fxp<+,52,14>)
    n203 = local read "Sin wave freq._y (Hz)"() -> (w446:fxp<+/-,32,6>)
    n204 = Multiply(x="Sin wave freq._y (Hz)", y=fxp<+/-,10,3> 2.0) -> (x*y=w454:fxp<+/-,41,9>)
    n205 = local read "Sin magnitude_y"() -> (w444:fxp<+/-,21,6>)
    n206 = local read "Sin magnitude_y"() -> (w437:fxp<+/-,21,6>)
    n207 = local read "Sin omega_y"() -> (w440:fxp<+/-,34,9>)
    n208 = Multiply(x=w454, y=w453) -> (x*y=w452:fxp<+/-,41,19>)
    n209 = Square(x=w440) -> (x^2=w439:fxp<+,34,18>)
    n210 = xnode "High Throughput Sine & Cosine"("x (pi)"=w452) -> ("sin(x)"=w434:fxp<+/-,16,2>, "cos(x)"=w442:fxp<+/-,16,2>)
    n211 = Multiply(x=w447, y=w446) -> (x*y=w445:fxp<+/-,34,9>)
    "Sin omega_y" <- w445
    n212 = Negate(x=w439) -> (-x=w438:fxp<+/-,35,19>)
    n213 = Multiply(x=w445, y=w444) -> (x*y=w443:fxp<+/-,33,15>)
    n214 = Multiply(x=w438, y=w437) -> (x*y=w436:fxp<+/-,34,20>)
    n215 = Multiply(x=w442, y=w443) -> (x*y=→"Dyr_sin_d":fxp<+/-,33,15>)
    n216 = Multiply(x="Sin magnitude_y", y=w434) -> (x*y=w450:fxp<+/-,37,8>)
    n217 = Multiply(x=w434, y=w436) -> (x*y=→"Dyr_sin_dd":fxp<+/-,35,20>)
    n218 = Add(x=w450, y="Sin offset_y") -> (x+y=→"Dyr_sin":fxp<+/-,37,8>)
    n219 = local read "Sin wave freq._p (Hz)"() -> (w411:fxp<+/-,32,6>)
    n220 = local read "Time now(s)"() -> (w429:fxp<+,52,14>)
    n221 = local read "Sin magnitude_p"() -> (w412:fxp<+/-,21,6>)
    n222 = local read "Sin magnitude_p"() -> (w414:fxp<+/-,21,6>)
    n223 = local read "Sin omega_p"() -> (w413:fxp<+/-,34,9>)
    n224 = Multiply(x="Sin wave freq._p (Hz)", y=fxp<+/-,10,3> 2.0) -> (x*y=w433:fxp<+/-,42,9>)
    n225 = Multiply(x=w433, y=w429) -> (x*y=w430:fxp<+/-,41,19>)
    n226 = Square(x=w413) -> (x^2=w425:fxp<+,34,18>)
    n227 = xnode "High Throughput Sine & Cosine"("x (pi)"=w430) -> ("sin(x)"=w416:fxp<+/-,16,2>, "cos(x)"=w421:fxp<+/-,16,2>)
    n228 = Multiply(x=w415, y=w411) -> (x*y=w428:fxp<+/-,34,9>)
    "Sin omega_p" <- w428
    n229 = Negate(x=w425) -> (-x=w424:fxp<+/-,35,19>)
    n230 = Multiply(x=w428, y=w412) -> (x*y=w427:fxp<+/-,33,15>)
    n231 = Multiply(x=w424, y=w414) -> (x*y=w423:fxp<+/-,35,19>)
    n232 = Multiply(x=w421, y=w427) -> (x*y=→"Dpr_sin_d":fxp<+/-,33,15>)
    n233 = Multiply(x=w416, y=w423) -> (x*y=→"Dpr_sin_dd":fxp<+/-,35,20>)
    n234 = Multiply(x="Sin magnitude_p", y=w416) -> (x*y=w419:fxp<+/-,37,8>)
    n235 = Add(x=w419, y="Sin offset_p") -> (x+y=→"Dpr_sin":fxp<+/-,37,8>)
  }
  n236 = while "Time reset" {
    shift-right: [w526] -> _
    shift-left: _ -> [w527]
    shift-right: [w521] -> _
    shift-left: _ -> [w522]
    stop <- FALSE stop-if-true
    n237 = local read "Stop motor_y"() -> (w528:bool)
    n238 = call "Tick Count3"() -> ("Tick Count(uSec)"=w526:u32)
    n239 = Subtract(x=w526, y=w527) -> (x-y=w525:u32)
    n240 = Add(x=w522, y=w525) -> (x+y=w524:u32)
    n241 = Select(t=u32 0, s=w528, f=w524) -> (s? t:f=w521:u32)
    n242 = To Fixed-Point(number=w521) -> (fixed-point=w520:fxp<+,32,32>)  [unwired: 1 in]
    n243 = Multiply(x=fxp<+,20,-18> 1.0000003385357559e-06, y=w520) -> (x*y=→"Time now(s)":fxp<+,52,14>)
  }
  n244 = while "Ini" {
    stop <- FALSE stop-if-true
    n245 = case shown="True" "Ini coe." {
      frame False {
      }
      frame True {
        w532 = T2 20 items=["50.000 kS/s (NI 9237)"=1, "25.000 kS/s (NI 9237)"=2, "16.667 kS/s (NI 9237)"=3, "12.500 kS/s (NI 9237)"=4, "10.000 kS/s (NI 9237)"=5, "8.333 kS/s (NI 9237)"=6, "7.143 kS/s (NI 9237)"=7, "6.250 kS/s (NI 9237)"=8, "5.556 kS/s (NI 9237)"=9, "5.000 kS/s (NI 9237)"=10, "4.545 kS/s (NI 9237)"=11, "4.167 kS/s (NI 9237)"=12, "3.846 kS/s (NI 9237)"=13, "3.571 kS/s (NI 9237)"=14, "3.333 kS/s (NI 9237)"=15, "3.125 kS/s (NI 9237)"=16, "2.941 kS/s (NI 9237)"=17, "2.778 kS/s (NI 9237)"=18, "2.632 kS/s (NI 9237)"=19, "2.500 kS/s (NI 9237)"=20, "2.381 kS/s (NI 9237)"=21, "2.273 kS/s (NI 9237)"=22, "2.174 kS/s (NI 9237)"=23, "2.083 kS/s (NI 9237)"=24, "2.000 kS/s (NI 9237)"=25, "1.923 kS/s (NI 9237)"=26, "1.852 kS/s (NI 9237)"=27, "1.786 kS/s (NI 9237)"=28, "1.724 kS/s (NI 9237)"=29, "1.667 kS/s (NI 9237)"=30, "1.613 kS/s (NI 9237)"=31] ("Data Rate")
        w549 = i16 0 items=["Step", "Sine"] ("Command_p")
        w550 = i16 2 items=["Raw", "Avg.", "Avg. w. filter"] ("Strain selection_p")
        w551 = i16 0 items=["Step", "Sine"] ("Command_y")
        w552 = i16 2 items=["Raw", "Avg.", "Avg. w. filter"] ("Strain selection_y")
        w554 = fxp<+/-,25,-10> 5.851034075021744e-07  # S/F coeff_p
        w553 = fxp<+/-,25,-10> 1.0477961041033268e-06  # S/F coeff_y
        w560 = i16 0 items=["Backward", "Forward"] ("Drive mode")
        n246 = local write "Sin wave freq._y (Hz)"(fxp<+/-,32,6> 1.0 ("Sin wave freq. (Hz)")) -> ()
        n247 = local write "Sin magnitude_y"(fxp<+/-,22,7> 5.0 ("Sin magnitude")) -> ()
        n248 = local write "fy_tolorance"(fxp<+,22,6> 5.0 ("f_tolorance")) -> ()
        n249 = local write "Sin offset_y"(fxp<+/-,38,9> 0.0 ("Sin offset")) -> ()
        n250 = local write "Dyr_step"(fxp<+/-,22,7> 0.0 ("Dr")) -> ()
        n251 = local write "Kp_y"(fxp<+/-,36,9> 30.0 ("Kp")) -> ()
        n252 = local write "Kd_y"(fxp<+/-,36,9> 0.0 ("Kd")) -> ()
        n253 = local write "Kv_y"(fxp<+/-,22,8> 0.0 ("Kv")) -> ()
        n254 = local write "Bv_y"(fxp<+/-,22,8> 0.0 ("Bv")) -> ()
        n255 = local write "Ki_y"(fxp<+/-,36,9> 0.0 ("Ki")) -> ()
        n256 = local write "S/F coeff_p"(w554) -> ()
        n257 = local write "S/F coeff_y"(w553) -> ()
        n258 = local write "Data Rate"(w532) -> ()
        n259 = local write "dFy_add"(FALSE ("dF_add")) -> ()
        n260 = local write "dFp_add"(FALSE ("dFp_add")) -> ()
        n261 = local write "Sin wave freq._p (Hz)"(fxp<+/-,32,6> 1.0 ("Sin wave freq._p (Hz)")) -> ()
        n262 = local write "Sin magnitude_p"(fxp<+/-,21,6> 5.0 ("Sin magnitude_p")) -> ()
        n263 = local write "fp_tolorance"(fxp<+,22,6> 5.0 ("fp_tolorance")) -> ()
        n264 = local write "Sin offset_p"(fxp<+/-,22,7> 0.0 ("Sin offset_p")) -> ()
        n265 = local write "Dpr_step"(fxp<+/-,22,7> 0.0 ("Dpr_step")) -> ()
        n266 = local write "Kp_p"(fxp<+/-,36,9> 30.0 ("Kp_p")) -> ()
        n267 = local write "Kd_p"(fxp<+/-,36,9> 0.0 ("Kd_p")) -> ()
        n268 = local write "Kv_p"(fxp<+/-,22,8> 0.0 ("Kv_p")) -> ()
        n269 = local write "Bv_p"(fxp<+/-,22,8> 0.0 ("Bv_p")) -> ()
        n270 = local write "Ki_p"(fxp<+/-,36,9> 0.0 ("Ki_p")) -> ()
        n271 = local write "Strain selection_p"(w550) -> ()
        n272 = local write "Strain selection_y"(w552) -> ()
        n273 = local write "Command_p"(w549) -> ()
        n274 = local write "Command_y"(w551) -> ()
        n275 = local write "Drive mode"(w560) -> ()
        n276 = local write "Dp_d_M_avg_Tc (uSec)"(u32 1000 ("D_d_M_avg_Tc (uSec)")) -> ()
        n277 = local write "Dy_d_M_avg_Tc (uSec)"(1000 ("Dy_d_M_avg_Tc (uSec)")) -> ()
        n278 = local write "Belt_out_p"(fxp<+/-,7,7> 22.0 ("Belt_op")) -> ()
        n279 = local write "Belt_out_y"(fxp<+/-,7,7> 22.0 ("Belt_oy")) -> ()
        n280 = local write "Belt_in_p"(fxp<+/-,6,6> 16.0 ("Belt_mp")) -> ()
        n281 = local write "Belt_in_y"(fxp<+/-,6,6> 16.0 ("Belt_my")) -> ()
      }
    }
  }
  n282 = while "FIFO" {
    stop <- FALSE stop-if-true
    n283 = flat-sequence {
      frame #0 {
        n284 = call "Loop Timer"("Count(uSec)"=u32 1000) -> ()  [unwired: 1 out]
      }
      frame #1 {
        n285 = local read "D_y(mm)"() -> (w586:fxp<+/-,32,7>)
        n286 = local read "Raw Strain_y"() -> (w585:fxp<+/-,36,4>)
        n287 = local read "Strain_y (Avg8)"() -> (w584:fxp<+/-,36,4>)
        n288 = local read "Strain_y (Avg8 w. f)"() -> (w583:fxp<+/-,36,8>)
        n289 = local read "Force_y"() -> (w579:fxp<+/-,32,10>)
        n290 = local read "Fy_dc"() -> (w581:fxp<+/-,32,10>)
        n291 = local read "D_p(mm)"() -> (w578:fxp<+/-,32,7>)
        n292 = local read "Raw Strain_p"() -> (w577:fxp<+/-,36,4>)
        n293 = local read "Strain_p (Avg8)"() -> (w576:fxp<+/-,36,4>)
        n294 = local read "Strain_p (Avg8 w. f)"() -> (w575:fxp<+/-,36,8>)
        n295 = local read "Force_p"() -> (w574:fxp<+/-,32,10>)
        n296 = local read "Dp_d (mm/s)"() -> (w573:fxp<+/-,36,13>)
        n297 = local read "Fp_dc"() -> (w572:fxp<+/-,32,10>)
        n298 = local read "Dy_d (T)"() -> (w580:fxp<+/-,36,13>)
        n299 = Build Array(w586, w585, w584, w583, w579, w580, w581, i16 0, w578, w577, w576, w575, w574, w573, w572, 0 ("element")) -> (w570:fxp<+/-,64,32>[])
        n300 = xnode ("FIFO Write")("Element"=w570, "Timeout"=0) -> ()  [unwired: 1 in, 2 out]
      }
    }
  }
  n301 = while "PID force controller_y" {
    stop <- FALSE stop-if-true
    n302 = local read "Force_y"() -> (w604:fxp<+/-,32,10>)
    n303 = local read "fyt_d"() -> (w588:fxp<+/-,36,18>)
    n304 = local read "Fr_y"() -> (w590:fxp<+/-,32,10>)
    n305 = xnode "High Throughput Subtract"("x"=w590, "y"=w604) -> ("x-y"=w603:fxp<+/-,33,11>)
    "fy_tilde" <- w603
    n306 = Absolute Value(x=w603) -> (abs(x)=w594:fxp<+,33,11>)
    n307 = local read "fyt_i"() -> (w589:fxp<+/-,36,16>)
    n308 = xnode ("High Throughput Multiply")("x"="Kp_y", "y"=w603) -> ("x*y"=w601:fxp<+/-,64,20>)
    n309 = xnode ("High Throughput Multiply")("x"="Kd_y", "y"=w588) -> ("x*y"=w600:fxp<+/-,64,27>)
    n310 = xnode ("High Throughput Add")("x"=w601, "y"=w600) -> ("x+y"=w597:fxp<+/-,64,28>)
    n311 = xnode ("High Throughput Multiply")("x"="Ki_y", "y"=w589) -> ("x*y"=w598:fxp<+/-,64,25>)
    n312 = Greater?(x=w594, y="fy_tolorance") -> (0:w592:bool)
    n313 = xnode ("High Throughput Add")("x"=w597, "y"=w598) -> ("x+y"=w596:fxp<+/-,64,29>)
    n314 = Select(t=w596, s=w592, f=fxp<+/-,51,14> 0.0) -> (s? t:f=→"Fy_PID":fxp<+/-,64,29>)
  }
  n315 = while {
    tunnel: w16 -> [w650]
    tunnel: [w624] -> w9
    shift-right: [w648] -> _
    shift-left: _ -> [w649]
    shift-right: [w644] -> _
    shift-left: _ -> [w645]
    shift-right: [w639] -> _
    shift-left: _ -> [w638]
    shift-right: [w638] -> _
    shift-left: _ -> [w637]
    shift-right: [w637] -> _
    shift-left: _ -> [w636]
    shift-right: [w636] -> _
    shift-left: _ -> [w635]
    shift-right: [w635] -> _
    shift-left: _ -> [w634]
    shift-right: [w634] -> _
    shift-left: _ -> [w633]
    shift-right: [w633] -> _
    shift-left: _ -> [w632]
    tunnel: w16 -> [w628]
    shift-right: [w621] -> _
    shift-left: _ -> [w622]
    shift-right: [w617] -> _
    shift-left: _ -> [w616]
    shift-right: [w616] -> _
    shift-left: _ -> [w615]
    shift-right: [w615] -> _
    shift-left: _ -> [w614]
    shift-right: [w614] -> _
    shift-left: _ -> [w613]
    shift-right: [w613] -> _
    shift-left: _ -> [w612]
    shift-right: [w612] -> _
    shift-left: _ -> [w611]
    shift-right: [w611] -> _
    shift-left: _ -> [w610]
    stop <- w625 stop-if-true
    w619 = fxp<+,20,2> 2.115001678466797  # Gage Factor
    n316 = xnode "FPGA I/O Node"("error in"=w650) -> ("error out"=w624:errorcluster, "Mod6/AI2"=w646:fxp<+/-,24,-4>)  [unwired: 1 in, 1 out]
    n317 = xnode "FPGA I/O Node"("error in"=w628) -> ("error out"=w626:errorcluster, "Mod6/AI3"=w620:fxp<+/-,24,-4>)  [unwired: 1 in, 1 out]
    n318 = Or(x=w624, y="Stop (Strain)") -> (x .or. y?=w627:bool)
    n319 = Select(t=w620, s="Strain gage reset_p", f=w622) -> (s? t:f=w621:fxp<+/-,24,-4>)
    n320 = Select(t=w646, s="Strain gage reset_y", f=w649) -> (s? t:f=w648:fxp<+/-,24,-4>)
    n321 = Or(x=w627, y=w626) -> (x .or. y?=w625:bool)
    n322 = Subtract(x=w620, y=w621) -> (x-y=w618:fxp<+/-,30,-3>)
    "Mod6/AI3" <- w618
    n323 = Subtract(x=w646, y=w648) -> (x-y=w647:fxp<+/-,30,-3>)
    "Mod6/AI2" <- w647
    n324 = Multiply(x=w619, y=w647) -> (x*y=w639:fxp<+/-,41,6>)
    "Raw Strain_y" <- w639
    n325 = Multiply(x=w619, y=w618) -> (x*y=w617:fxp<+/-,50,-1>)
    "Raw Strain_p" <- w617
    n326 = call "average_v2.vi"("Numeric 8"=w610, "Numeric"=w617, "Numeric 7"=w611, "Numeric 2"=w616, "Numeric 6"=w612, "Numeric 5"=w613, "Numeric 4"=w614, "Numeric 3"=w615) -> ("Mean (8pt)"=w609:fxp<+/-,32,4>)  [unwired: 1 in, 2 out]
    "Strain_p (Avg8)" <- w609
    n327 = call "average_v2.vi"("Numeric 8"=w632, "Numeric"=w639, "Numeric 7"=w633, "Numeric 2"=w638, "Numeric 6"=w634, "Numeric 5"=w635, "Numeric 4"=w636, "Numeric 3"=w637) -> ("Mean (8pt)"=w631:fxp<+/-,32,4>)  [unwired: 1 in, 2 out]
    "Strain_y (Avg8)" <- w631
    n328 = call "Tick Count"() -> ("Tick Count(uSec)"=w644:u32)
    n329 = xnode "Butterworth Filter"("input data"=w609, "scaled coefficients"="Strain_p Avg.8 coeff.") -> ("output data"=→"Strain_p (Avg8 w. f)":fxp<+/-,36,8>)  [unwired: 1 in]
    n330 = xnode "Butterworth Filter"("input data"=w631, "scaled coefficients"="Strain_y Avg8 coeff.") -> ("output data"=→"Strain_y (Avg8 w. f)":fxp<+/-,32,4>)  [unwired: 1 in]
    n331 = Subtract(x=w644, y=w645) -> (x-y=w642:fxp<+/-,32,16>)
    n332 = Divide(x=fxp<+,7,10> 1000.0, y=w642) -> (x/y=→"Loop rate (kHz)":fxp<+/-,40,27>)
  }
  n333 = for {
    N: w5 -> [_]
    tunnel: [w669] -> w4 mode=indexing
    tunnel: [w668] -> w3 mode=indexing
    tunnel: ["Dy_d_M_avg_Tc (uSec)"] -> w2
    n334 = local read "Encoder Position_y"() -> (w668:i32)
    n335 = call "Wait3"("Count(uSec)"="Dy_d_M_avg_Tc (uSec)") -> ("Tick Count(uSec)"=w669:u32)
  }
  n336 = for {
    N: w8 -> [_]
    tunnel: ["Dp_d_M_avg_Tc (uSec)"] -> w1
    tunnel: [w671] -> w7 mode=indexing
    tunnel: [w670] -> w6 mode=indexing
    n337 = local read "Encoder Position_p"() -> (w670:i32)
    n338 = call "Wait2"("Count(uSec)"="Dp_d_M_avg_Tc (uSec)") -> ("Tick Count(uSec)"=w671:u32)
  }
  n339 = while "Omega_y (Mavg)" {
    tunnel: w5 -> [w696]
    shift-right: [w694] -> _
    shift-left: w4 -> [w699]
    shift-right: [w693] -> _
    shift-left: w3 -> [w695]
    shift-right: [w688] -> _
    shift-left: _ -> [w692]
    tunnel: w2 -> [w687]
    stop <- FALSE stop-if-true
    w675 = fxp<+/-,32,0> 0.3183098859153688  # L/2/pi
    w684 = fxp<+,32,0> 0.1953125  # 800/4096
    w690 = fxp<+/-,27,3> 0.007853984832763672  # 2*pi/800
    n340 = call "Tick Count6"() -> ("Tick Count(uSec)"=w700:u32)
    n341 = Index Array(array=w699, index=0) -> (element=w698:u32)
    n342 = Index Array(array=w695, index=0) -> (element=w697:i32)
    n343 = Multiply(x=w696, y=w687) -> (x*y=w702:i32)
    n344 = Add(x=w702, y=w698) -> (x+y=w701:u32)
    n345 = Greater Or Equal?(x=w700, y=w701) -> (x >= y?=w691:bool)
    n346 = case shown="True" w691 {
      tunnel: w700 -> [_ w723]
      tunnel: w696 -> [_ w720]
      tunnel: w699 -> [w707 w722]
      tunnel: w698 -> [_ w721]
      tunnel: w697 -> [_ w717]
      tunnel: w695 -> [w706 w719]
      tunnel: [w705 w715] -> w688
      tunnel: [w707 w714] -> w694
      tunnel: [w706 w713] -> w693
      tunnel: w692 -> [w705 _]
      frame False {
      }
      frame True {
        # "count/s"
        n347 = local read "Encoder Position_y"() -> (w716:i32)
        n348 = Subtract(x=w723, y=w721) -> (x-y=w724:u32)
        n349 = Insert Into Array(array=w722, new element=w723) -> (w726:u32[])  [unwired: 1 in]
        n350 = Subtract(x=w716, y=w717) -> (x-y=w711:i32)
        n351 = Insert Into Array(array=w719, index=w720, new element=w716) -> (w727:i32[])
        n352 = To Fixed-Point(number=w724) -> (fixed-point=w710:fxp<+,32,32>)  [unwired: 1 in]
        n353 = To Fixed-Point(number=w711) -> (fixed-point=w718:fxp<+/-,32,32>)  [unwired: 1 in]
        n354 = Divide(x=w710, y=fxp<+,32,32> 1000000.0) -> (x/y=w709:fxp<+,64,32>)
        n355 = Delete From Array(array=w726, length=1, index=0) -> (array with subset deleted=w714:u32[])  [unwired: 1 out]
        n356 = Delete From Array(array=w727, length=1, index=0) -> (array with subset deleted=w713:i32[])  [unwired: 1 out]
        n357 = Divide(x=w718, y=w709) -> (x/y=w715:fxp<+/-,40,20>)
      }
    }
    n358 = local read "Mag. factor_p"() -> (w683:fxp<+/-,20,3>)
    n359 = local read "Mag. encoder_y"() -> (w686:bool)
    n360 = local read "Belt_in_y"() -> (w677:fxp<+/-,6,6>)
    n361 = Multiply(x=w690, y=w688) -> (x*y=w680:fxp<+/-,40,14>)
    n362 = Divide(x=w684, y=w683) -> (x/y=w682:fxp<+/-,53,18>)
    n363 = local read "Belt_out_y"() -> (w678:fxp<+/-,7,7>)
    n364 = Select(t=w682, s=w686, f=fxp<+,1,1> 1.0) -> (s? t:f=w681:fxp<+/-,53,18>)
    n365 = Multiply(x=w675, y=w677) -> (x*y=w676:fxp<+/-,38,6>)
    n366 = Multiply(x=w681, y=w680) -> (x*y=w679:fxp<+/-,36,14>)
    "omega_y (Mavg)" <- w679
    n367 = Divide(x=w676, y=w678) -> (x/y=w674:fxp<+/-,45,6>)
    n368 = Multiply(x=w674, y=w679) -> (x*y=→"Dy_d (Mavg)":fxp<+/-,36,14>)
  }
  n369 = while "Omega_p (Mavg)" {
    tunnel: w8 -> [w753]
    shift-right: [w751] -> _
    shift-left: w7 -> [w756]
    shift-right: [w750] -> _
    shift-left: w6 -> [w752]
    shift-right: [w749] -> _
    shift-left: _ -> [w748]
    tunnel: w1 -> [w746]
    stop <- FALSE stop-if-true
    w735 = fxp<+/-,27,3> 0.007853984832763672  # 2*pi/800
    w737 = fxp<+,32,0> 0.1953125  # 800/4096
    w734 = fxp<+/-,32,0> 0.3183098859153688  # L/2/pi
    n370 = call "Tick Count5"() -> ("Tick Count(uSec)"=w757:u32)
    n371 = Index Array(array=w756, index=0) -> (element=w755:u32)
    n372 = Index Array(array=w752, index=0) -> (element=w754:i32)
    n373 = Multiply(x=w753, y=w746) -> (x*y=w759:i32)
    n374 = Add(x=w759, y=w755) -> (x+y=w758:u32)
    n375 = Greater Or Equal?(x=w757, y=w758) -> (x >= y?=w747:bool)
    n376 = case shown="True" w747 {
      tunnel: w757 -> [_ w780]
      tunnel: w753 -> [_ w777]
      tunnel: w756 -> [w764 w779]
      tunnel: w755 -> [_ w778]
      tunnel: w754 -> [_ w774]
      tunnel: w752 -> [w763 w776]
      tunnel: [w762 w772] -> w749
      tunnel: [w764 w771] -> w751
      tunnel: [w763 w770] -> w750
      tunnel: w748 -> [w762 _]
      frame False {
      }
      frame True {
        n377 = local read "Encoder Position_p"() -> (w773:i32)
        n378 = Subtract(x=w780, y=w778) -> (x-y=w781:u32)
        n379 = Subtract(x=w773, y=w774) -> (x-y=w765:i32)
        n380 = Insert Into Array(array=w779, new element=w780) -> (w783:u32[])  [unwired: 1 in]
        n381 = Insert Into Array(array=w776, index=w777, new element=w773) -> (w784:i32[])
        n382 = To Fixed-Point(number=w781) -> (fixed-point=w767:fxp<+,32,32>)  [unwired: 1 in]
        n383 = To Fixed-Point(number=w765) -> (fixed-point=w775:fxp<+/-,32,32>)  [unwired: 1 in]
        n384 = Delete From Array(array=w783, length=1, index=0) -> (array with subset deleted=w771:u32[])  [unwired: 1 out]
        n385 = Delete From Array(array=w784, length=1, index=0) -> (array with subset deleted=w770:i32[])  [unwired: 1 out]
        n386 = Divide(x=w767, y=fxp<+,32,32> 1000000.0) -> (x/y=w768:fxp<+,64,32>)
        n387 = Divide(x=w775, y=w768) -> (x/y=w772:fxp<+/-,40,20>)
      }
    }
    n388 = local read "Mag. factor_p"() -> (w738:fxp<+/-,20,3>)
    n389 = local read "Mag. encoder_p"() -> (w745:bool)
    n390 = local read "Belt_in_p"() -> (w742:fxp<+/-,6,6>)
    n391 = Divide(x=w737, y=w738) -> (x/y=w736:fxp<+/-,53,18>)
    n392 = local read "Belt_out_p"() -> (w741:fxp<+/-,7,7>)
    n393 = Multiply(x=w735, y=w749) -> (x*y=w743:fxp<+/-,40,14>)
    n394 = Select(t=w736, s=w745, f=fxp<+/-,52,3> 1.0) -> (s? t:f=w730:fxp<+/-,64,18>)
    n395 = Multiply(x=w734, y=w742) -> (x*y=w740:fxp<+/-,38,6>)
    n396 = Multiply(x=w730, y=w743) -> (x*y=w733:fxp<+/-,36,14>)
    "omega_p (Mavg)" <- w733
    n397 = Divide(x=w740, y=w741) -> (x/y=w732:fxp<+/-,45,6>)
    n398 = Multiply(x=w732, y=w733) -> (x*y=→"Dp_d (Mavg)":fxp<+/-,36,14>)
  }
  n399 = while "Quadrature drive_p" {
    stop <- FALSE stop-if-true
    n400 = local read "dFp_PID"() -> (w788:fxp<+/-,36,18>)
    n401 = local read "omega_p (rad/s)"() -> (w794:fxp<+/-,36,13>)
    n402 = local read "Fp_PID"() -> (w789:fxp<+/-,36,16>)
    n403 = Select(t=w788, s="dFp_add", f=fxp<+,1,1> 0.0) -> (s? t:f=w792:fxp<+/-,36,18>)
    n404 = call "Oriental_step_motor_PKP225.vi"("F_Threshold"=fxp<+,12,12> 10.0, "dFmr"=w792, "omega"=w794, "Fmr"=w789) -> ("vq_F"=→"vq_p_F":fxp<+/-,20,5>, "vd_F"=→"vd_p_F":fxp<+/-,20,5>)  [unwired: 6 in]
  }
  n405 = while "PID force controller_p" {
    stop <- FALSE stop-if-true
    n406 = local read "Force_p"() -> (w809:fxp<+/-,32,10>)
    n407 = local read "fpt_d"() -> (w800:fxp<+/-,36,18>)
    n408 = local read "Fr_p"() -> (w810:fxp<+/-,32,10>)
    n409 = xnode "High Throughput Subtract"("x"=w810, "y"=w809) -> ("x-y"=w801:fxp<+/-,33,11>)
    "fp_tilde" <- w801
    n410 = local read "fpt_i"() -> (w798:fxp<+/-,34,18>)
    n411 = xnode ("High Throughput Multiply")("x"="Kp_p", "y"=w801) -> ("x*y"=w799:fxp<+/-,64,20>)
    n412 = xnode ("High Throughput Multiply")("x"="Kd_p", "y"=w800) -> ("x*y"=w815:fxp<+/-,64,27>)
    n413 = Absolute Value(x=w801) -> (abs(x)=w808:fxp<+,33,11>)
    n414 = xnode ("High Throughput Add")("x"=w799, "y"=w815) -> ("x+y"=w813:fxp<+/-,64,28>)
    n415 = xnode ("High Throughput Multiply")("x"="Ki_p", "y"=w798) -> ("x*y"=w814:fxp<+/-,64,27>)
    n416 = xnode ("High Throughput Add")("x"=w813, "y"=w814) -> ("x+y"=w804:fxp<+/-,64,29>)
    n417 = Greater?(x=w808, y="fp_tolorance") -> (0:w805:bool)
    n418 = Select(t=w804, s=w805, f=fxp<+,1,1> 0.0) -> (s? t:f=→"Fp_PID":fxp<+/-,64,29>)
  }
  n419 = while "PD position controller_p" {
    stop <- FALSE stop-if-true
    n420 = local read "Drive mode"() -> (w818:i16)
    n421 = case shown="1" w818 {
      tunnel: [fxp<+/-,62,19> 0.0 w821] -> w817
      frame 0, Default {
        # "Backward"
      }
      frame 1 {
        # "Forward"
        n422 = local read "D_p(mm)"() -> (w828:fxp<+/-,32,7>)
        n423 = local read "Dp_error_d"() -> (w820:fxp<+/-,33,8>)
        n424 = local read "Dpr_for"() -> (w827:fxp<+/-,22,7>)
        n425 = Subtract(x=w827, y=w828) -> (x-y=w826:fxp<+/-,24,8>)
        "Dp_error" <- w826
        n426 = Multiply(x=w826, y="Kv_p") -> (x*y=w823:fxp<+/-,34,16>)
        n427 = Multiply(x=w820, y="Bv_p") -> (x*y=w822:fxp<+/-,55,16>)
        n428 = Add(x=w823, y=w822) -> (x+y=w821:fxp<+/-,56,17>)
      }
    }
    "Fr_p" <- w817
  }
  n429 = while "All switch" {
    stop <- FALSE stop-if-true
    n430 = case shown="True" "Encoder reset" {
      frame False {
        n431 = local write "Encoder reset_p"(FALSE ("Encoder reset_p")) -> ()
        n432 = local write "Encoder reset_y"(FALSE ("Encoder reset_y")) -> ()
      }
      frame True {
        n433 = flat-sequence {
          frame #0 {
            n434 = local write "Encoder reset_p"(TRUE ("Encoder reset_p")) -> ()
          }
          frame #1 {
            n435 = local write "Encoder reset_y"(TRUE ("Encoder reset_y")) -> ()
            n436 = local write "Encoder reset_p"(FALSE ("Encoder reset_p")) -> ()
          }
          frame #2 {
            n437 = local write "Encoder reset_y"(FALSE ("Encoder reset_y")) -> ()
          }
        }
      }
    }
  }
  n438 = while "Derivative" {
    stop <- FALSE stop-if-true
    n439 = local read "Dpr_sin_dd"() -> (w845:fxp<+/-,35,20>)
    n440 = local read "Stop motor_y"() -> (w851:bool)
    n441 = local read "Dyr_sin_dd"() -> (w853:fxp<+/-,35,20>)
    n442 = local read "Dpr_sin_d"() -> (w847:fxp<+/-,33,15>)
    n443 = local read "Stop motor_p"() -> (w843:bool)
    n444 = local read "Dyr_sin_d"() -> (w856:fxp<+/-,33,15>)
    n445 = local read "Dp_error"() -> (w848:fxp<+/-,22,7>)
    n446 = local read "Dy_error"() -> (w857:fxp<+/-,22,7>)
    n447 = local read "Dp_dd"() -> (w846:fxp<+/-,36,25>)
    n448 = local read "Dy_dd"() -> (w854:fxp<+/-,36,25>)
    n449 = Subtract(x=w856, y=w857) -> (x-y=w855:fxp<+/-,34,16>)
    n450 = Subtract(x=w853, y=w854) -> (x-y=w852:fxp<+/-,41,26>)
    n451 = Subtract(x=w847, y=w848) -> (x-y=w840:fxp<+/-,34,16>)
    n452 = Subtract(x=w845, y=w846) -> (x-y=w844:fxp<+/-,41,26>)
    n453 = Select(t=fxp<+,1,1> 0.0, s=w851, f=w855) -> (s? t:f=→"Dy_error_d":fxp<+/-,34,16>)
    n454 = Select(t=fxp<+/-,64,49> 0.0, s=w851, f=w852) -> (s? t:f=→"Dy_error_dd":fxp<+/-,64,49>)
    n455 = Select(t=fxp<+,1,1> 0.0, s=w843, f=w840) -> (s? t:f=→"Dp_error_d":fxp<+/-,34,16>)
    n456 = Select(t=fxp<+/-,41,26> 0.0, s=w843, f=w844) -> (s? t:f=→"Dp_error_dd":fxp<+/-,41,26>)
  }
  n457 = while "ft_d" {
    stop <- FALSE stop-if-true
    n458 = local read "Dy_error_dd"() -> (w875:fxp<+/-,36,16>)
    n459 = local read "Dp_error_dd"() -> (w866:fxp<+/-,36,16>)
    n460 = local read "Dy_error_d"() -> (w877:fxp<+/-,33,8>)
    n461 = local read "Dp_error_d"() -> (w868:fxp<+/-,33,8>)
    n462 = local read "Kv_p"() -> (w869:fxp<+/-,22,8>)
    n463 = local read "Bv_p"() -> (w867:fxp<+/-,22,8>)
    n464 = local read "Kv_y"() -> (w878:fxp<+/-,22,8>)
    n465 = local read "Bv_y"() -> (w876:fxp<+/-,22,8>)
    n466 = local read "Force_y"() -> (w871:fxp<+/-,32,10>)
    n467 = Multiply(x=w877, y=w878) -> (x*y=w873:fxp<+/-,55,16>)
    n468 = Multiply(x=w875, y=w876) -> (x*y=w874:fxp<+/-,58,24>)
    n469 = Multiply(x=w868, y=w869) -> (x*y=w864:fxp<+/-,55,16>)
    n470 = Multiply(x=w866, y=w867) -> (x*y=w865:fxp<+/-,58,24>)
    n471 = local read "Force_p"() -> (w862:fxp<+/-,32,10>)
    n472 = Add(x=w873, y=w874) -> (x+y=w872:fxp<+/-,63,24>)
    n473 = Add(x=w864, y=w865) -> (x+y=w863:fxp<+/-,63,24>)
    n474 = Subtract(x=w872, y=w871) -> (x-y=→"fyt_d":fxp<+/-,63,24>)
    n475 = Subtract(x=w863, y=w862) -> (x-y=→"fpt_d":fxp<+/-,63,24>)
  }
  n476 = while "Encoder_y" {
    shift-right: [w917] -> _
    shift-left: _ -> [w909]
    shift-right: [w916] -> _
    shift-left: _ -> [w908]
    shift-right: [w907] -> _
    shift-left: _ -> [w905]
    shift-right: [w913] -> _
    shift-left: _ -> [w910]
    shift-right: [w912] -> _
    shift-left: _ -> [w911]
    shift-right: [w906] -> _
    shift-left: _ -> [w904]
    stop <- FALSE stop-if-true
    w887 = fxp<+/-,16,1> 0.0244140625  # 2*50/4096
    w894 = fxp<+/-,20,-5> 0.00048828125  # L/4096
    w899 = fxp<+/-,20,-5> 0.002499997615814209  # L/800
    w903 = fxp<+/-,16,1> 0.125  # 2*50/800
    n477 = xnode "FPGA I/O Node"() -> ("Mod7/DIO2"=w918:bool, "Mod7/DIO3"=w919:bool)  [unwired: 2 in, 2 out]
    n478 = xnode "FPGA I/O Node"() -> ("Mod7/DIO6"=w915:bool, "Mod7/DIO7"=w914:bool)  [unwired: 2 in, 2 out]
    n479 = local read "Encoder reset_y"() -> (w879:bool)
    n480 = call "encoder_sub.vi"("A_pre"=w909, "B_pre"=w908, "Encoder Position_pre"=w905, "A input"=w918, "Encoder Position Reset"="Encoder reset_y", "B input"=w919) -> ("A"=w917:bool, "B"=w916:bool, "Encoder Position (Counts)"=w907:i32)  [unwired: 19 in]
    "Encoder Position_y1" <- w907
    n481 = call "encoder_sub.vi"("A_pre"=w910, "B_pre"=w911, "Encoder Position_pre"=w904, "A input"=w915, "Encoder Position Reset"=w879, "B input"=w914) -> ("A"=w913:bool, "B"=w912:bool, "Encoder Position (Counts)"=w906:i32)  [unwired: 19 in]
    "Encoder Position_y2" <- w906
    n482 = local read "Belt_in_y"() -> (w892:fxp<+/-,6,6>)
    n483 = local read "Belt_in_y"() -> (w898:fxp<+/-,6,6>)
    n484 = local read "Belt_out_y"() -> (w890:fxp<+/-,7,7>)
    n485 = Divide(x=w894, y="Mag. factor_y") -> (x/y=w893:fxp<+/-,32,0>)
    n486 = local read "Belt_out_y"() -> (w897:fxp<+/-,7,7>)
    n487 = To Fixed-Point(number=w906) -> (fixed-point=w888:fxp<+/-,21,21>)  [unwired: 1 in]
    n488 = local read "Mag. factor_y"() -> (w886:fxp<+/-,20,3>)
    n489 = To Fixed-Point(number=w907) -> (fixed-point=w902:fxp<+/-,16,16>)  [unwired: 1 in]
    n490 = Multiply(x=w893, y=w892) -> (x*y=w891:fxp<+/-,32,6>)
    n491 = Multiply(x=w899, y=w898) -> (x*y=w901:fxp<+/-,26,1>)
    n492 = Divide(x=w891, y=w890) -> (x/y=w889:fxp<+/-,36,6>)
    n493 = Divide(x=w901, y=w897) -> (x/y=w900:fxp<+/-,27,2>)
    n494 = Divide(x=w887, y=w886) -> (x/y=w885:fxp<+/-,20,0>)
    n495 = xnode "High Throughput Multiply"("x"=w889, "y"=w888) -> ("x*y"=→"D_y2":fxp<+/-,57,27>)
    n496 = xnode "High Throughput Multiply"("x"=w902, "y"=w903) -> ("x*y"=→"rad_y1":fxp<+/-,32,17>)
    n497 = xnode "High Throughput Multiply"("x"=w888, "y"=w885) -> ("x*y"=→"rad_y2":fxp<+/-,41,21>)
    n498 = xnode "High Throughput Multiply"("x"=w900, "y"=w902) -> ("x*y"=→"D_y1":fxp<+/-,43,18>)
  }
  n499 = while "Omega_y(T method)" {
    shift-right: [w946] -> _
    shift-left: _ -> [w947]
    shift-right: [w931] -> _
    shift-left: _ -> [w949]
    shift-right: [w951] -> _
    shift-left: _ -> [w952]
    shift-right: [w938] -> _
    shift-left: _ -> [w936]
    shift-right: [w930] -> _
    shift-left: _ -> [w937]
    shift-right: [w934] -> _
    shift-left: _ -> [w935]
    stop <- FALSE stop-if-true
    w928 = fxp<+/-,32,0> 0.3183098859153688  # L/2/pi
    w940 = fxp<+,32,0> 0.1953125  # 800/4096
    w945 = fxp<+/-,32,0> 0.3183098859153688  # L/2/pi
    n500 = local read "Encoder Position_y1"() -> (w946:i32)
    n501 = call "Tick Count2"() -> ("Tick Count(Ticks)"=w932:u32)
    n502 = local read "Encoder Position_y2"() -> (w938:i32)
    n503 = local read "Mag. factor_y"() -> (w939:fxp<+/-,20,3>)
    n504 = call "omega_sub_Encoder_800ppr.vi"("mt0"="mt0_omega_y", "omega_pre"=w949, "ticks_m_pre"=w952, "ticks"=w932, "count_pre"=w947, "count"=w946) -> ("ticks_m"=w951:u32, "mt"=→"mt_omega_y1":u32, "omega"=w931:fxp<+/-,36,13>)  [unwired: 3 in]
    "omega_y1 (T)" <- w931
    n505 = call "omega_sub_Encoder_800ppr.vi"("omega_pre"=w937, "ticks_m_pre"=w935, "ticks"=w932, "count_pre"=w936, "count"=w938) -> ("ticks_m"=w934:u32, "mt"=→"mt_omega_y2":u32, "omega"=w930:fxp<+/-,36,13>)  [unwired: 4 in]
    n506 = local read "Belt_in_y"() -> (w927:fxp<+/-,6,6>)
    n507 = local read "Belt_out_y"() -> (w925:fxp<+/-,7,7>)
    n508 = Divide(x=w940, y=w939) -> (x/y=w929:fxp<+/-,53,18>)
    n509 = Multiply(x=w945, y="Belt_in_y") -> (x*y=w943:fxp<+/-,38,6>)
    n510 = Multiply(x=w928, y=w927) -> (x*y=w926:fxp<+/-,38,6>)
    n511 = Divide(x=w926, y=w925) -> (x/y=w924:fxp<+/-,45,6>)
    n512 = Divide(x=w943, y="Belt_out_y") -> (x/y=w941:fxp<+/-,20,1>)
    n513 = Multiply(x=w930, y=w929) -> (x*y=w923:fxp<+/-,64,30>)
    "omega_y2 (T)" <- w923
    n514 = xnode ("High Throughput Multiply")("x"=w924, "y"=w923) -> ("x*y"=→"Dy2_d (T)":fxp<+/-,64,36>)
    n515 = xnode ("High Throughput Multiply")("x"=w941, "y"=w931) -> ("x*y"=→"Dy1_d (T)":fxp<+/-,56,14>)
  }
  n516 = xnode "FPGA I/O Node"("error in"=w9, "Mod6/Stop"=TRUE) -> ()  [unwired: 1 in, 2 out]
  n517 = while {
    stop <- FALSE stop-if-true
    n518 = case shown="True" "Set 3" {
      frame False {
      }
      frame True {
        n519 = local write "fp_tolorance"(fxp<+,22,6> 3.0 ("fp_tolorance")) -> ()
        n520 = local write "Kp_p"(fxp<+/-,36,9> 100.0 ("Kp_p")) -> ()
      }
    }
    n521 = case shown="True" "Set 2" {
      frame False {
      }
      frame True {
        n522 = local write "fp_tolorance"(fxp<+,22,6> 1.5 ("fp_tolorance")) -> ()
        n523 = local write "Kp_p"(fxp<+/-,36,9> 50.0 ("Kp_p")) -> ()
      }
    }
    n524 = case shown="True" "Set 1" {
      frame False {
      }
      frame True {
        n525 = local write "fp_tolorance"(fxp<+,22,6> 3.0 ("fp_tolorance")) -> ()
        n526 = local write "Kp_p"(fxp<+/-,36,9> 50.0 ("Kp_p")) -> ()
      }
    }
    n527 = case shown="True" "Set 5" {
      frame False {
      }
      frame True {
        n528 = local write "fp_tolorance"(fxp<+,22,6> 3.0 ("fp_tolorance")) -> ()
        n529 = local write "Kp_p"(fxp<+/-,36,9> 150.0 ("Kp_p")) -> ()
      }
    }
    n530 = case shown="True" "Set 6" {
      frame False {
      }
      frame True {
        n531 = local write "fp_tolorance"(fxp<+,22,6> 1.5 ("fp_tolorance")) -> ()
        n532 = local write "Kp_p"(fxp<+/-,36,9> 150.0 ("Kp_p")) -> ()
      }
    }
    n533 = case shown="True" "Set 4" {
      frame False {
      }
      frame True {
        n534 = local write "fp_tolorance"(fxp<+,22,6> 1.5 ("fp_tolorance")) -> ()
        n535 = local write "Kp_p"(fxp<+/-,36,9> 100.0 ("Kp_p")) -> ()
      }
    }
  }
